vi "Curtin_PlaySound.vi"(8 "Task":enum16{"play", "save"}(ring), 10 "all waveforms":waveform(dbl)[](array[waveform]), 11 "device ID":u32) -> (0 "error out":errorcluster)   [LabVIEW 2022 SP3]
uses:
  <vilib>/sound2/lvsound2.llb/Sound Output Write Simple (DBL2).vi
panel:
  in  "Timeout (sec)":dbl=-1.0
  in  "Resolution (bits)":i32=16
  out "Waveform Graph":waveform(dbl)[](graph)
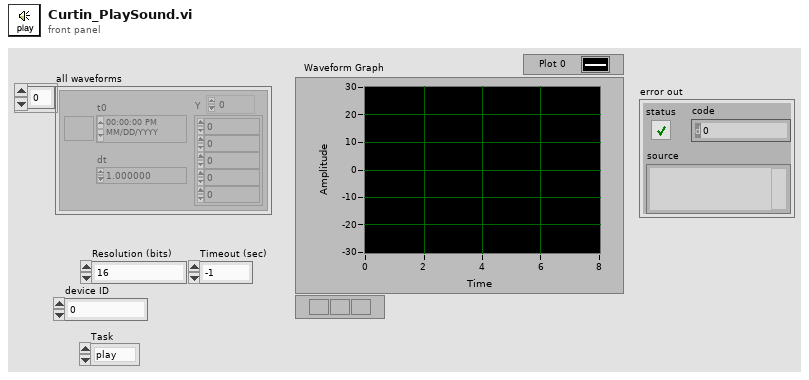
[diagram p1: front panel]
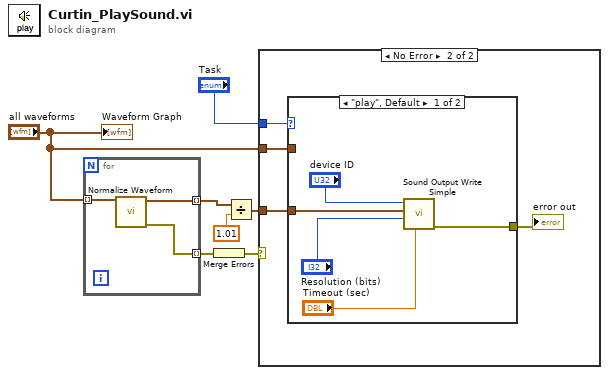
[diagram p0: block diagram]
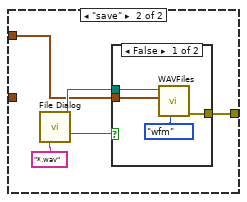
[diagram p3: hidden frame]
diagram:
  n1 = for {
    tunnel: "all waveforms" -> [w9] mode=indexing
    tunnel: [w10] -> w6 mode=indexing
    tunnel: [w8] -> w2 mode=indexing
    n2 = call <vilib>:"Normalize Waveform.vi"("waveform in"=w9) -> ("error out"=w8:errorcluster, "normalized waveform"=w10:waveform(dbl))  [unwired: 7 in, 2 out]
  }
  n3 = Merge Errors(w2) -> (w1:errorcluster)
  n4 = Divide(x=w6, y=1.01 ("scale")) -> (x/y=w7:waveform(dbl)[])
  n5 = case shown="No Error" w1 {
    tunnel: w7 -> [_ w14]
    tunnel: "Task" -> [_ w13]
    tunnel: "all waveforms" -> [_ w11]
    frame Error {
    }
    frame No Error {
      n6 = case shown="\"play\", Default" w13 {
        tunnel: w14 -> [w19 _]
        tunnel: [w18 w24] -> w12
        tunnel: w11 -> [_ w20]
        frame "play", Default {
          n7 = call-poly <vilib>:"Sound Output Write Simple.vi"("timeout (sec)"="Timeout (sec)", "bits per sample"="Resolution (bits)", "data"=w19, "device ID"="device ID") -> ("error out"=w18:errorcluster)  [unwired: 7 in]
        }
        frame "save" {
          n8 = call "File Dialog"("pattern (all files)"="*.wav" ("pattern label")) -> ("selected path"=w22:path, "cancelled"=w21:bool)  [unwired: 11 in, 2 out]
          n9 = case shown="False" w21 {
            tunnel: w20 -> [w27 _]
            tunnel: [w26 _] -> w24
            tunnel: w22 -> [w25 _]
            frame False {
              n10 = call "WAVFiles.vi"("Task"=enum16{"Read", "Write", "wfm"}."wfm", "Wfm data"=w27, "WAV File"=w25) -> ("error out"=w26:errorcluster)  [unwired: 5 in, 3 out]
            }
            frame True {
            }
          }
        }
      }
      "error out" <- w12
    }
  }
  "Waveform Graph" <- "all waveforms"
